vi "Advance Control Mode.vi"(8 "error in (no error)":errorcluster, 10 "Gripper Command":T1={"Finger A"={"Position"=0, "Speed"=255, "Force"=255}, "Finger B"={"Position"=0, "Speed"=255, "Force"=255}, "Finger C"={"Position"=0, "Speed"=255, "Force"=255}, "Scissor"={"Position"=0, "Speed"=255, "Force"=255}}, 11 "Robotiq in":refnum<class "Robotiq.lvclass">) -> (0 "error out":errorcluster, 3 "Robotiq out":refnum<class "Robotiq.lvclass">)   [LabVIEW 2011, in "Robotiq.lvclass"]
uses:
  Robotiq.lvclass
  Controls/Gripper Command.ctl
  Controls/Finger Command.ctl
  Robotiq.lvclass/Robotiq.ctl
  <vilib>/NI Modbus.llb/MB Ethernet Master Query Write Multiple Registers (poly).vi
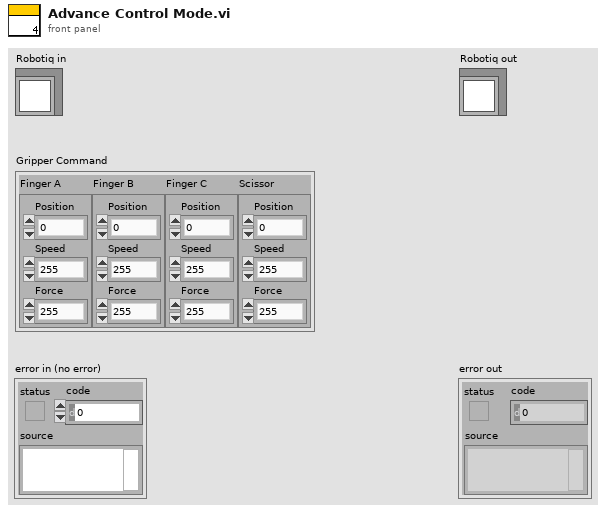
[diagram p1: front panel]
types:
  T1 = typedef "Gripper Command.ctl" = cluster{"Finger A":T2, "Finger B":T2, "Finger C":T2, "Scissor":T2}
  T2 = typedef "Finger Command.ctl" = cluster{"Position":u8, "Speed":u8, "Force":u8}
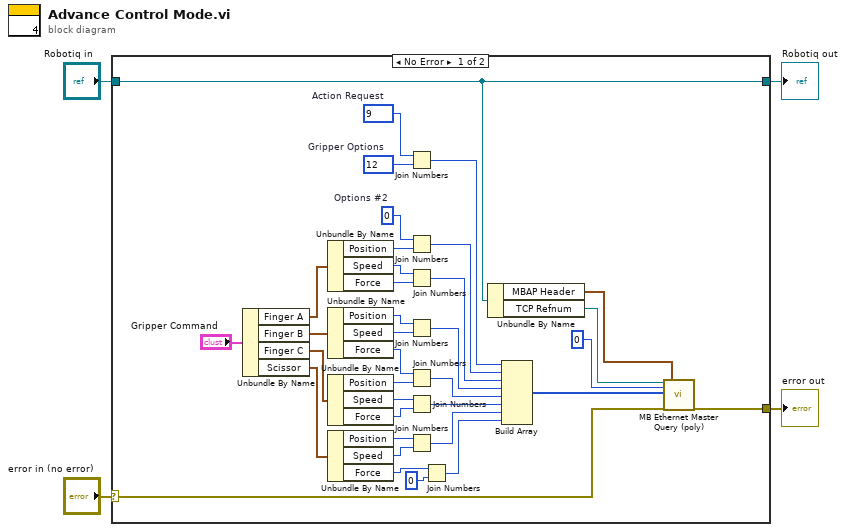
[diagram p0: block diagram]
diagram:
  n1 = case shown="No Error" "error in (no error)" {
    selector: "error in (no error)" -> [w9 w42]
    tunnel: [w8 w42] -> w3
    tunnel: [w40 w41] -> w1
    tunnel: "Robotiq in" -> [w40 w41]
    frame No Error {
      w7 = u8 9  # Action Request
      w27 = u8 0  # Options #2
      w6 = u8 12  # Gripper Options
      n2 = Unbundle By Name("Gripper Command") -> ("Finger A"=w26:T2, "Finger B"=w18:T2, "Finger C"=w14:T2, "Scissor"=w10:T2)
      n3 = Unbundle By Name(w26) -> ("Position"=w24:u8, "Speed"=w23:u8, "Force"=w22:u8)
      n4 = Unbundle By Name(w18) -> ("Position"=w21:u8, "Speed"=w20:u8, "Force"=w19:u8)
      n5 = Unbundle By Name(w14) -> ("Position"=w15:u8, "Speed"=w16:u8, "Force"=w17:u8)
      n6 = Unbundle By Name(w10) -> ("Position"=w13:u8, "Speed"=w12:u8, "Force"=w11:u8)
      n7 = Join Numbers(hi=w7, lo=w6) -> ((hi.lo)=w5:u16)
      n8 = Join Numbers(hi=w27, lo=w24) -> ((hi.lo)=w28:u16)
      n9 = Join Numbers(hi=w23, lo=w22) -> ((hi.lo)=w36:u16)
      n10 = Join Numbers(hi=w21, lo=w20) -> ((hi.lo)=w35:u16)
      n11 = Join Numbers(hi=w19, lo=w15) -> ((hi.lo)=w34:u16)
      n12 = Join Numbers(hi=w16, lo=w17) -> ((hi.lo)=w33:u16)
      n13 = Join Numbers(hi=w13, lo=w12) -> ((hi.lo)=w32:u16)
      n14 = Join Numbers(hi=w11, lo=u8 0 ("Speed")) -> ((hi.lo)=w31:u16)
      n15 = Unbundle By Name(w40) -> ("MBAP Header"=w39:cluster{"Transaction ID":u16, "Unit ID":u8}, "TCP Refnum"=w38:refnum<k5>)
      n16 = Build Array(w5, w28, w36, w35, w34, w33, w32, w31) -> (w30:u16[])
      n17 = call-poly <vilib>:"MB Ethernet Master Query (poly).vi"("TCP Connection Refnum in"=w38, "Starting Address"=u16 0 ("Address"), "Registers"=w30, "error in"=w9, "MBAP Header"=w39) -> ("error out"=w8:errorcluster)  [unwired: 12 in, 2 out]
    }
    frame Error {
    }
  }
  "error out" <- w3
  "Robotiq out" <- w1
